vi "Combo2.vi"   [LabVIEW 2016, in "Test.lvrbt"]
uses:
  Test.lvrbt
  <vilib>/NXT/Block Support/NXT_InputPort.ctl
  <vilib>/NXT/Subs/ColorSensorColors.ctl
  <vilib>/NXT/Hardware/Plugins/Tetrix DC Motor/TetrixDCMotorAddress.ctl
  <vilib>/NXT/Hardware/Plugins/Tetrix 180 deg Servo/Tetrix180ServoAddress.ctl
  <vilib>/NXT/NXTIO Xnodes/NXTIONodeSubVIs/TETRIX IO Move Servos.vi
  <vilib>/NXT/Dual Mode Library/Waits/Wait_Num.vi
  <vilib>/NXT/NXTIO Xnodes/NXTIONodeSubVIs/TETRIX IO Move DC Motors.vi
  <vilib>/NXT/Dual Mode Library/Waits/Wait_EV3_Ultrasonic_Centimeter_Closer.vi
  <vilib>/NXT/NXTIO Xnodes/NXTIONodeSubVIs/TETRIX IO Stop DC Motors.vi
  <vilib>/NXT/Dual Mode Library/Waits/Wait_EV3_Ultrasonic_Centimeters_Further.vi
  <vilib>/NXT/Dual Mode Library/Waits/Wait_EV3_Color_Color.vi
  <vilib>/NXT/NXTIO Xnodes/AddressXNode/NXTIOAddress.xnode
  <vilib>/NXT/Subs/LVHSConnector.ctl
  <vilib>/NXT/NXTIO Xnodes/NXTIOXNode/NXTIO.xnode
  <vilib>/NXT/LegoClasses/BrickReference/BrickReference.lvclass
types:
  T1 = typedef "NXT_InputPort.ctl" = u32
  T2 = typedef "ColorSensorColors.ctl" = enum16{"No Color", "Black", "Blue", "Green", "Yellow", "Red", "White", "Brown"}
  T3 = typedef "Tetrix180ServoAddress.ctl" = i32
  T4 = cluster{"Tetrix180Servo":T3, "Tetrix180Servo":T3, "Tetrix180Servo":T3, "Tetrix180Servo":T3, "Tetrix180Servo":T3}
  T5 = typedef "LVHSConnector.ctl" = refnum<class "BrickReference.lvclass">
  T6 = typedef "TetrixDCMotorAddress.ctl" = i32
diagram:
  w6 = T1 2 items=["Port 1", "Port 2", "Port 3", "Port 4"] ("Port (Port 1)")
  w77 = T1 1 items=["Port 1", "Port 2", "Port 3", "Port 4"] ("Port (Port 1)")
  w116 = T1 1 items=["Port 1", "Port 2", "Port 3", "Port 4"] ("Port (Port 1)")
  w120 = T1 1 items=["Port 1", "Port 2", "Port 3", "Port 4"] ("Port (Port 1)")
  w121 = T1 1 items=["Port 1", "Port 2", "Port 3", "Port 4"] ("Port (Port 1)")
  # "Function 6:\n\nRelease the first ball"
  n1 = xnode "Motors"() -> ("Motor"=w99:T4)
  n2 = xnode "Move Servos"("Position 5"=u8 200, "Position 4"=u8 40, "Position 3"=u8 0, "Position 2"=u8 0, "Position 1"=u8 242, "Motors"=w99) -> ("NXT/EV3"=w95:T5)  [unwired: 1 in]
  n3 = xnode "Motors"() -> ("Motor"=w133:cluster{"TetrixDCMotor":T6, "TetrixDCMotor":T6})
  n4 = call-poly <vilib>:"PolyWait.vi"("Time (1 sec)"=sgl 1.0, "NXT/EV3"=w95) -> ("NXT/EV3"=w94:T5)  [unwired: 2 in]
  n5 = xnode "Move Motors"("Power/Speed 2"=i8 100, "Power/Speed 1"=i8 100, "Motors"=w133, "NXT/EV3"=w94) -> ("NXT/EV3"=w136:T5)
  n6 = call-poly <vilib>:"PolyWait.vi"("Centimeters (40)"=sgl 6.5, "NXT/EV3"=w136, "Port (Port 1)"=w121) -> ("NXT/EV3"=w134:T5)  [unwired: 1 in]
  n7 = xnode "Stop Motors"("Motors"=w133, "NXT/EV3"=w134) -> ("NXT/EV3"=w132:T5)
  n8 = xnode "Motors"() -> ("Motor"=w124:cluster{"TetrixDCMotor":T6, "TetrixDCMotor":T6})
  n9 = call-poly <vilib>:"PolyWait.vi"("Time (1 sec)"=sgl 1.0, "NXT/EV3"=w132) -> ("NXT/EV3"=w130:T5)  [unwired: 2 in]
  n10 = xnode "Move Motors"("Power/Speed 2"=i8 20, "Power/Speed 1"=i8 21, "Motors"=w124, "NXT/EV3"=w130) -> ("NXT/EV3"=w127:T5)
  n11 = call-poly <vilib>:"PolyWait.vi"("Centimeters (50)"=sgl 5.0, "NXT/EV3"=w127, "Port (Port 1)"=w120) -> ("NXT/EV3"=w125:T5)  [unwired: 1 in]
  n12 = xnode "Stop Motors"("Motors"=w124, "NXT/EV3"=w125) -> ("NXT/EV3"=w122:T5)
  n13 = xnode "Motors"() -> ("Motor"=w83:cluster{"TetrixDCMotor":T6, "TetrixDCMotor":T6})
  n14 = call-poly <vilib>:"PolyWait.vi"("Time (1 sec)"=sgl 1.0, "NXT/EV3"=w122) -> ("NXT/EV3"=w78:T5)  [unwired: 2 in]
  n15 = xnode "Move Motors"("Power/Speed 2"=i8 -5, "Power/Speed 1"=i8 -5, "Motors"=w83, "NXT/EV3"=w78) -> ("NXT/EV3"=w85:T5)
  n16 = call-poly <vilib>:"PolyWait.vi"("Centimeters (40)"=sgl 5.0, "NXT/EV3"=w85, "Port (Port 1)"=w77) -> ("NXT/EV3"=w84:T5)  [unwired: 1 in]
  n17 = xnode "Stop Motors"("Motors"=w83, "NXT/EV3"=w84) -> ("NXT/EV3"=w72:T5)
  n18 = xnode "Motors"() -> ("Motor"=w68:cluster{"TetrixDCMotor":T6, "TetrixDCMotor":T6})
  n19 = call-poly <vilib>:"PolyWait.vi"("Time (1 sec)"=sgl 1.0, "NXT/EV3"=w72) -> ("NXT/EV3"=w73:T5)  [unwired: 2 in]
  n20 = xnode "Move Motors"("Power/Speed 2"=i8 5, "Power/Speed 1"=i8 5, "Motors"=w68, "NXT/EV3"=w73) -> ("NXT/EV3"=w70:T5)
  n21 = call-poly <vilib>:"PolyWait.vi"("Time (1 sec)"=sgl 0.6, "NXT/EV3"=w70) -> ("NXT/EV3"=w67:T5)  [unwired: 2 in]
  n22 = xnode "Stop Motors"("Motors"=w68, "NXT/EV3"=w67) -> ("NXT/EV3"=w69:T5)
  n23 = call-poly <vilib>:"PolyWait.vi"("Time (1 sec)"=sgl 1.0, "NXT/EV3"=w69) -> ("NXT/EV3"=w81:T5)  [unwired: 2 in]
  n24 = xnode "Motors"() -> ("Motor"=w111:T3)
  n25 = xnode "Move Servos"("Position 1"=u8 85, "Motors"=w111, "NXT/EV3"=w81) -> ("NXT/EV3"=w108:T5)
  n26 = call-poly <vilib>:"PolyWait.vi"("Time (1 sec)"=sgl 7.0, "NXT/EV3"=w108) -> ("NXT/EV3"=w105:T5)  [unwired: 2 in]
  n27 = xnode "Motors"() -> ("Motor"=w107:T3)
  n28 = xnode "Move Servos"("Position 1"=u8 227, "Motors"=w107, "NXT/EV3"=w105) -> ("NXT/EV3"=w103:T5)
  n29 = call-poly <vilib>:"PolyWait.vi"("Time (1 sec)"=sgl 0.5, "NXT/EV3"=w103) -> ("NXT/EV3"=w100:T5)  [unwired: 2 in]
  n30 = xnode "Motors"() -> ("Motor"=w102:T3)
  n31 = xnode "Move Servos"("Position 1"=u8 20, "Motors"=w102, "NXT/EV3"=w100) -> ("NXT/EV3"=w92:T5)
  n32 = call-poly <vilib>:"PolyWait.vi"("Time (1 sec)"=sgl 1.5, "NXT/EV3"=w92) -> ("NXT/EV3"=w89:T5)  [unwired: 2 in]
  n33 = xnode "Motors"() -> ("Motor"=w90:T3)
  n34 = xnode "Move Servos"("Position 1"=u8 98, "Motors"=w90, "NXT/EV3"=w89) -> ("NXT/EV3"=w88:T5)
  n35 = xnode "Motors"() -> ("Motor"=w114:cluster{"TetrixDCMotor":T6, "TetrixDCMotor":T6})
  n36 = call-poly <vilib>:"PolyWait.vi"("Time (1 sec)"=sgl 1.0, "NXT/EV3"=w88) -> ("NXT/EV3"=w112:T5)  [unwired: 2 in]
  n37 = xnode "Move Motors"("Power/Speed 2"=i8 5, "Power/Speed 1"=i8 5, "Motors"=w114, "NXT/EV3"=w112) -> ("NXT/EV3"=w117:T5)
  n38 = call-poly <vilib>:"PolyWait.vi"("Centimeters (50)"=sgl 5.0, "NXT/EV3"=w117, "Port (Port 1)"=w116) -> ("NXT/EV3"=w115:T5)  [unwired: 1 in]
  n39 = xnode "Stop Motors"("Motors"=w114, "NXT/EV3"=w115) -> ("NXT/EV3"=w65:T5)
  n40 = call-poly <vilib>:"PolyWait.vi"("Time (1 sec)"=sgl 1.0, "NXT/EV3"=w65) -> ("NXT/EV3"=w62:T5)  [unwired: 2 in]
  n41 = xnode "Motors"() -> ("Motor"=w63:T3)
  n42 = xnode "Move Servos"("Position 1"=u8 67, "Motors"=w63, "NXT/EV3"=w62) -> ("NXT/EV3"=w60:T5)
  n43 = call-poly <vilib>:"PolyWait.vi"("Time (1 sec)"=sgl 1.0, "NXT/EV3"=w60) -> ("NXT/EV3"=w57:T5)  [unwired: 2 in]
  n44 = xnode "Motors"() -> ("Motor"=w58:T3)
  n45 = xnode "Move Servos"("Position 1"=u8 240, "Motors"=w58, "NXT/EV3"=w57) -> ("NXT/EV3"=w52:T5)
  n46 = xnode "Motors"() -> ("Motor"=w45:cluster{"TetrixDCMotor":T6, "TetrixDCMotor":T6})
  n47 = call-poly <vilib>:"PolyWait.vi"("Time (1 sec)"=sgl 1.0, "NXT/EV3"=w52) -> ("NXT/EV3"=w51:T5)  [unwired: 2 in]
  n48 = xnode "Move Motors"("Power/Speed 2"=i8 -100, "Power/Speed 1"=i8 -100, "Motors"=w45, "NXT/EV3"=w51) -> ("NXT/EV3"=w47:T5)
  n49 = call-poly <vilib>:"PolyWait.vi"("Time (1 sec)"=sgl 1.0, "NXT/EV3"=w47) -> ("NXT/EV3"=w46:T5)  [unwired: 2 in]
  n50 = xnode "Stop Motors"("Motors"=w45, "NXT/EV3"=w46) -> ("NXT/EV3"=w43:T5)
  n51 = xnode "Motors"() -> ("Motor"=w36:cluster{"TetrixDCMotor":T6, "TetrixDCMotor":T6})
  n52 = call-poly <vilib>:"PolyWait.vi"("Time (1 sec)"=sgl 1.0, "NXT/EV3"=w43) -> ("NXT/EV3"=w40:T5)  [unwired: 2 in]
  n53 = xnode "Move Motors"("Power/Speed 2"=i8 -100, "Power/Speed 1"=i8 -100, "Motors"=w36, "NXT/EV3"=w40) -> ("NXT/EV3"=w38:T5)
  n54 = call-poly <vilib>:"PolyWait.vi"("Time (1 sec)"=sgl 1.0, "NXT/EV3"=w38) -> ("NXT/EV3"=w37:T5)  [unwired: 2 in]
  n55 = xnode "Stop Motors"("Motors"=w36, "NXT/EV3"=w37) -> ("NXT/EV3"=w34:T5)
  n56 = call-poly <vilib>:"PolyWait.vi"("Time (1 sec)"=sgl 1.0, "NXT/EV3"=w34) -> ("NXT/EV3"=w31:T5)  [unwired: 2 in]
  n57 = xnode "Motors"() -> ("Motor"=w32:T3)
  n58 = xnode "Move Servos"("Position 1"=u8 0, "Motors"=w32, "NXT/EV3"=w31) -> ("NXT/EV3"=w29:T5)
  n59 = call-poly <vilib>:"PolyWait.vi"("Time (1 sec)"=sgl 1.0, "NXT/EV3"=w29) -> ("NXT/EV3"=w26:T5)  [unwired: 2 in]
  n60 = xnode "Motors"() -> ("Motor"=w27:T3)
  n61 = xnode "Move Servos"("Position 1"=u8 242, "Motors"=w27, "NXT/EV3"=w26) -> ("NXT/EV3"=w24:T5)
  n62 = call-poly <vilib>:"PolyWait.vi"("Time (1 sec)"=sgl 1.0, "NXT/EV3"=w24) -> ("NXT/EV3"=w21:T5)  [unwired: 2 in]
  n63 = xnode "Motors"() -> ("Motor"=w22:T3)
  n64 = xnode "Move Servos"("Position 1"=u8 0, "Motors"=w22, "NXT/EV3"=w21) -> ("NXT/EV3"=w12:T5)
  n65 = xnode "Motors"() -> ("Motor"=w4:cluster{"TetrixDCMotor":T6, "TetrixDCMotor":T6})
  n66 = call-poly <vilib>:"PolyWait.vi"("Time (1 sec)"=sgl 1.5, "NXT/EV3"=w12) -> ("NXT/EV3"=w11:T5)  [unwired: 2 in]
  n67 = xnode "Move Motors"("Power/Speed 2"=i8 10, "Power/Speed 1"=i8 10, "Motors"=w4, "NXT/EV3"=w11) -> ("NXT/EV3"=w8:T5)
  n68 = call-poly <vilib>:"PolyWait.vi"("Color (Red)"=ColorSensorColors."Black", "NXT/EV3"=w8, "Port (Port 1)"=w6) -> ("NXT/EV3"=w5:T5)  [unwired: 1 in]
  n69 = xnode "Stop Motors"("Motors"=w4, "NXT/EV3"=w5) -> ("NXT/EV3"=w2:T5)
  n70 = call-poly <vilib>:"PolyWait.vi"("Time (1 sec)"=sgl 1.5, "NXT/EV3"=w2) -> ("NXT/EV3"=w1:T5)  [unwired: 2 in]
  n71 = xnode "Motors"() -> ("Motor"=w19:T3)
  n72 = xnode "Move Servos"("Position 1"=u8 118, "Motors"=w19, "NXT/EV3"=w1) -> ("NXT/EV3"=w17:T5)
  n73 = call-poly <vilib>:"PolyWait.vi"("Time (1 sec)"=sgl 2.0, "NXT/EV3"=w17) -> ("NXT/EV3"=w14:T5)  [unwired: 2 in]
  n74 = xnode "Motors"() -> ("Motor"=w15:T3)
  n75 = xnode "Move Servos"("Position 1"=u8 40, "Motors"=w15, "NXT/EV3"=w14) -> ()  [unwired: 1 out]
